vi "take_step.vi"(6 "Speed (um/s)":i32, 8 "error in (no error)":errorcluster, 9 "x,y,z step size (nm)":i32[](array[numeric]), 10 "device ID":i32, 11 "Handle in":i64) -> (0 "error out":errorcluster, 2 "Return (<0 is error)":i32, 3 "Handle out":i64)   [LabVIEW 2016, in "OSB_uMp_library.lvlib"]
doc: "Make uMp step by the specified amount (in nm).\n\nAll axes are moved simultaneously. Note that you could modify this VI to perform a move with independent x,y,z speeds.\n\nx,y,z step size (nm) should be an array with three elements, representing x, y, and z values.\nVI returns custom error code -8005 on the LabVIEW error cluster if the array is of the wrong length."
uses:
  OSB_uMp_library.lvlib
  <vilib>/Analysis/baseanly.llb/Unit Vector (DBL).vi
  ump.dll
  <vilib>/Analysis/NI_AALBase.lvlib
panel:
  # "By Stuart Box at OxSyBio Ltd, 2017\n\nThis software is provided WITHOUT ANY WARRANTY; without even the implied warranty of MERCHANTABILITY or FITNESS FOR A PARTICULAR PURPOSE.\n\ninfo@oxsybio.com\n\nOxSyBio Ltd, The Walbrook Building, 25 Walbrook, London, EC4N 8AF"
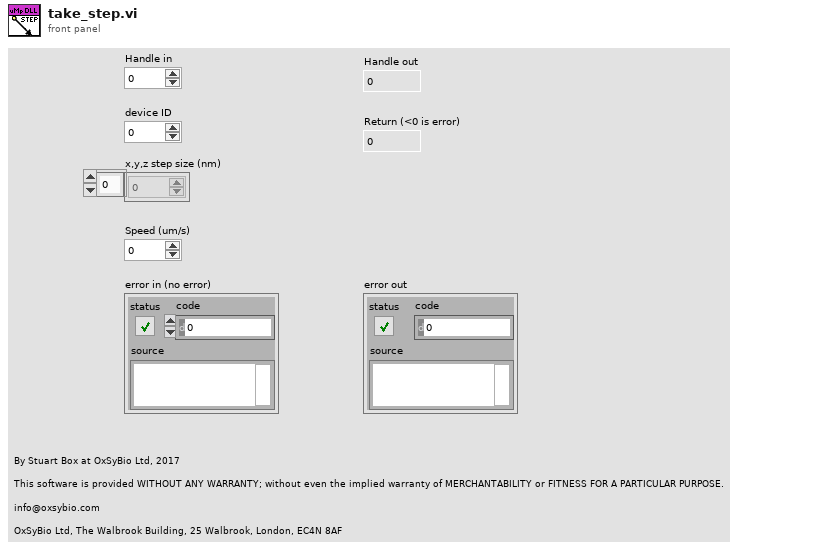
[diagram p1: front panel]
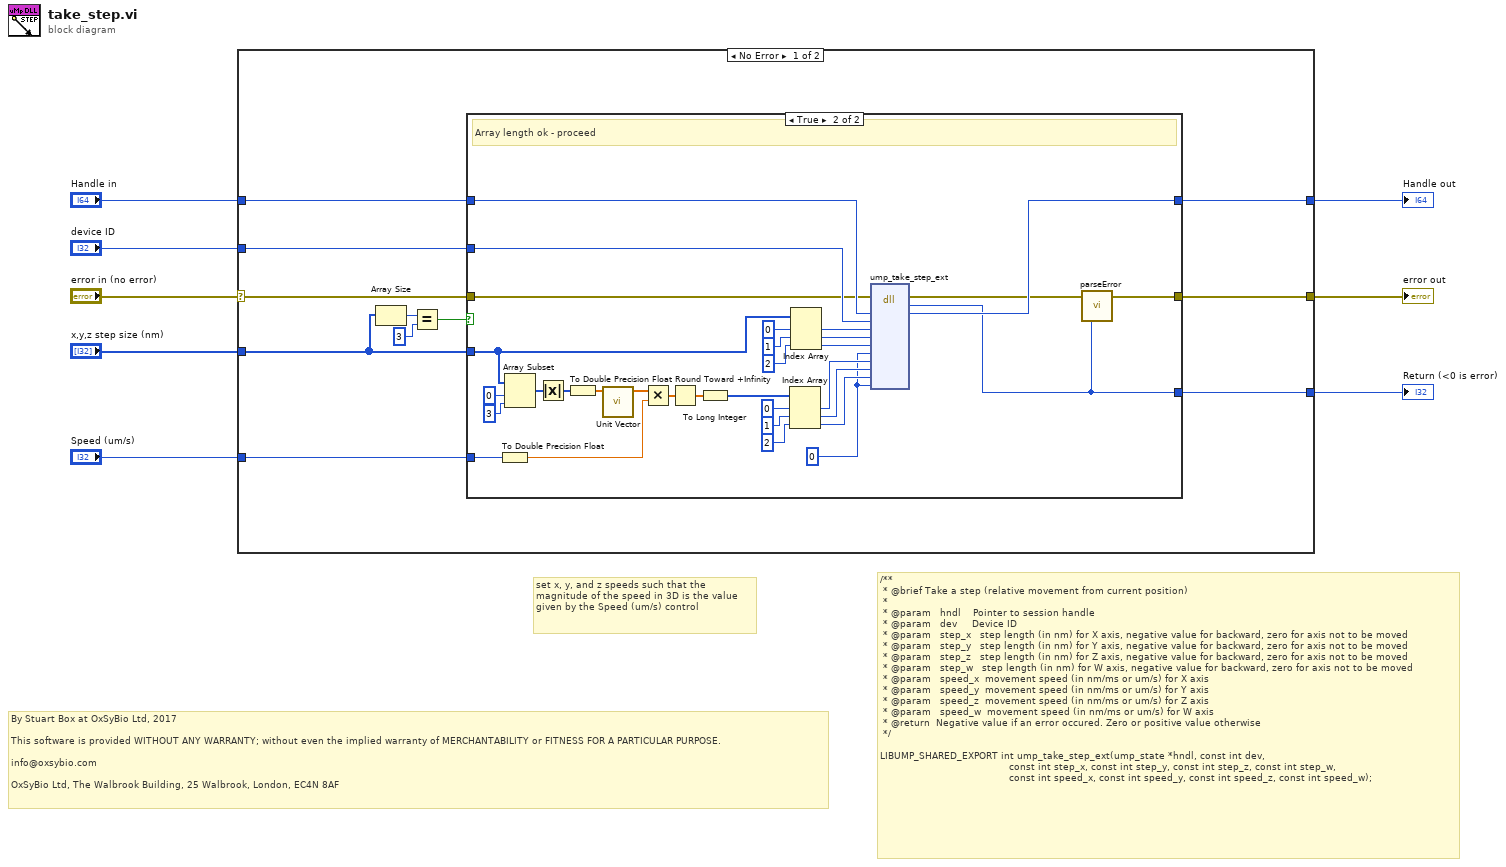
[diagram p0: block diagram]
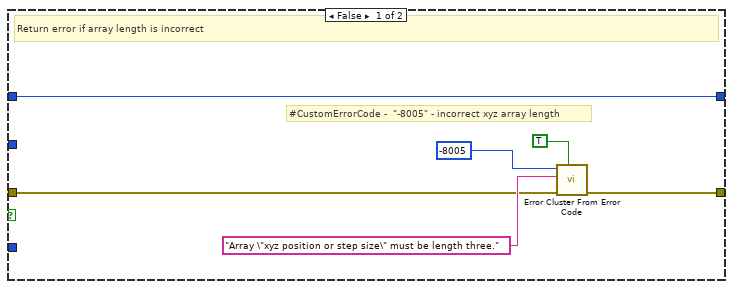
[diagram p2: hidden frame]
diagram:
  # "By Stuart Box at OxSyBio Ltd, 2017\n\nThis software is provided WITHOUT ANY WARRANTY; without even the implied warranty of MERCHANTABILITY or FITNESS FOR A PARTICULAR PURPOSE.\n\ninfo@oxsybio.com\n\nOxSyBio Ltd, The Walbrook Building, 25 Walbrook, London, EC4N 8AF"
  # "set x, y, and z speeds such that the magnitude of the speed in 3D is the value given by the Speed (um/s) control"
  # "/**\n * @brief Take a step (relative movement from current position)\n *\n * @param   hndl    Pointer to session handle\n * @param   dev     Device ID\n * @param   step_x   step length (in nm) for X axis, negative value for backward, zero for axis not to be moved\n * @param   step_y   step length (in nm) for Y axis, negative value for backward, zero for axis not to be moved\n * @param   step_z   step length (in nm) for Z axis, negative value for backward, zero for axis not to be moved\n * @param   step_w   step length (in nm) for W axis, negative value for backward, zero for axis not to be moved\n * @param   speed_x  movement speed (in nm/ms or um/s) for X axis\n * @param   speed_y  movement speed (in nm/ms or um/s) for Y axis\n * @param   speed_z  movement speed (in nm/ms or um/s) for Z axis\n * @param   speed_w  movement speed (in nm/ms or um/s) for W axis\n * @return  Negative value if an error occured. Zero or positive value otherwise\n */\n\nLIBUMP_SHARED_EXPORT int ump_take_step_ext(ump_state *hndl, const int dev,\n                                           const int step_x, const int step_y, const int step_z, const int step_w,\n                                           const int speed_x, const int speed_y, const int speed_z, const int speed_w);"
  n1 = case shown="No Error" "error in (no error)" {
    selector: "error in (no error)" -> [w13 w59]
    tunnel: "x,y,z step size (nm)" -> [w10 _]
    tunnel: "Speed (um/s)" -> [w19 _]
    tunnel: "device ID" -> [w18 _]
    tunnel: "Handle in" -> [w17 w58]
    tunnel: [w16 _] -> w4
    tunnel: [w15 w59] -> w3
    tunnel: [w14 w58] -> w2
    frame No Error {
      n2 = Array Size(array=w10) -> (size(s)=w11:i32)
      n3 = Equal?(x=w11, y=3) -> (x = y?=w9:bool)
      n4 = case shown="True" w9 {
        tunnel: w10 -> [_ w44]
        tunnel: w19 -> [_ w43]
        tunnel: w18 -> [_ w54]
        tunnel: w17 -> [w20 w53]
        tunnel: [_ w26] -> w16
        tunnel: [w21 w27] -> w15
        tunnel: [w20 w49] -> w14
        tunnel: w13 -> [w22 w48]
        frame False {
          # "#CustomErrorCode -  \"-8005\" - incorrect xyz array length"
          # "Return error if array length is incorrect"
          n5 = call <vilib>:"Error Cluster From Error Code.vi"("show call chain? (False)"=TRUE, "error in (no error)"=w22, "error message (\"\")"="Array \"xyz position or step size\" must be length three." ("error message (\"\")"), "error code (0)"=-8005) -> ("error out"=w21:errorcluster)  [unwired: 5 in]
        }
        frame True {
          w31 = 0 ("w")
          # "Array length ok - proceed"
          n6 = To Double Precision Float(number=w43) -> (double precision float=w42:dbl)
          n7 = Array Subset(array=w44, index=0, length=3) -> (w30:i32[])
          n8 = Absolute Value(x=w30) -> (abs(x)=w29:i32[])
          n9 = To Double Precision Float(number=w29) -> (double precision float=w45:dbl[])
          n10 = call-poly <vilib>:"Unit Vector.vi"("Input Vector"=w45) -> ("Unit Vector"=w41:dbl[])  [unwired: 8 in, 2 out]
          n11 = Multiply(x=w41, y=w42) -> (x*y=w40:dbl[])
          n12 = Round Toward +Infinity(x=w40) -> (ceil(x): smallest int >= x=w33:dbl[])
          n13 = To Long Integer(number=w33) -> (32bit integer=w32:i32[])
          n14 = Index Array(array=w32, index #1=0 ("index"), index #2=1 ("index"), index #3=2 ("index")) -> (element #1=w36:i32, element #2=w35:i32, element #3=w34:i32)
          n15 = Index Array(array=w44, index #1=0 ("index"), index #2=1 ("index"), index #3=2 ("index")) -> (element #1=w52:i32, element #2=w51:i32, element #3=w50:i32)
          n16 = dll-call lib="C:/Users/Stu/Desktop/OSB LabVIEW uMp/uMp_library/ump.dll" fn="ump_take_step_ext"(error in=w48, "handle"=w53, "devID"=w54, "x"=w52, "y"=w51, "z"=w50, "w"=w31, "speed_x"=w36, "speed_y"=w35, "speed_z"=w34, "speed_w"=w31) -> (error out=w28:errorcluster, "return"=w26:i32, "handle"=w49:i64)  [unwired: 11 in, 1 out]
          n17 = call "parseError.vi"("Error In"=w28, "ump dll return value (<0 is error)"=w26) -> ("Error Out"=w27:errorcluster)  [unwired: 24 in, 1 out]
        }
      }
    }
    frame Error {
    }
  }
  "Return (<0 is error)" <- w4
  "error out" <- w3
  "Handle out" <- w2
